vi "Clip ends.vi"(10 "Clip length":i32, 11 "Input":dbl[](array[numeric])) -> (3 "Output":dbl[](array[numeric]))   [LabVIEW 2018]
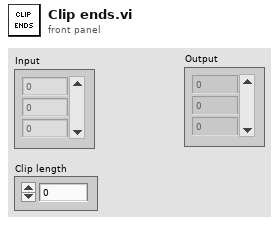
[diagram p1: front panel]
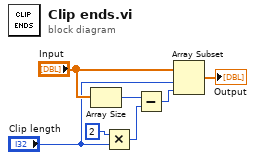
[diagram p0: block diagram]
diagram:
  n1 = Array Size(array="Input") -> (size(s)=w5:i32)
  n2 = Multiply(x=2, y="Clip length") -> (x*y=w2:i32)
  n3 = Subtract(x=w5, y=w2) -> (x-y=w1:i32)
  n4 = Array Subset(array="Input", index="Clip length", length=w1) -> (→"Output":dbl[])
